vi "Find STM connection by ID.vi"(8 "error in":errorcluster, 10 "Message ID":i32, 11 "STM connections":T1[](array[typedef])) -> (0 "error out":errorcluster, 3 "Connection Ref":T1)   [LabVIEW 2019, in "RemoteControl.STM.lvclass"]
uses:
  RemoteControl.STM.lvclass
  <vilib>/NI/STM/NI STM.lvlib
  <vilib>/NI/STM/TCP/Get Connection Reference (TCP).vi
  <vilib>/NI/STM/SubVIs/MetaDataElement.ctl
  <vilib>/NI/STM/TCP/TCP Connection Info.ctl
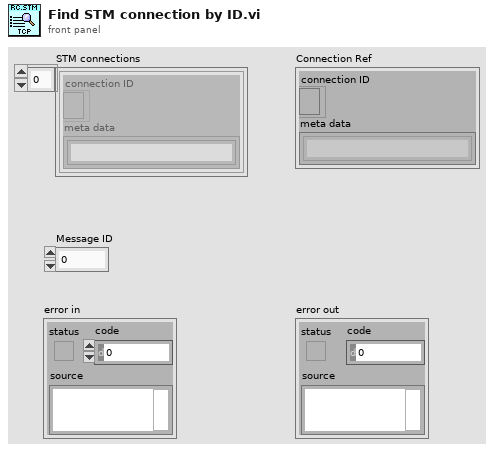
[diagram p1: front panel]
types:
  T1 = typedef "NI STM.lvlib/TCP Connection Info.ctl" = cluster{"connection ID":refnum<k5>, "meta data":T2[]}
  T2 = typedef "NI STM.lvlib/MetaDataElement.ctl" = string
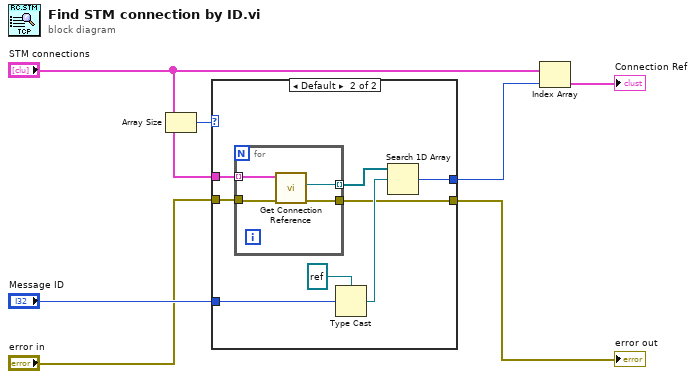
[diagram p0: block diagram]
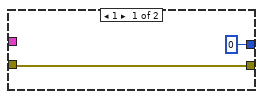
[diagram p2: hidden frame]
diagram:
  n1 = Array Size(array="STM connections") -> (size(s)=w4:i32)
  n2 = case shown="Default" w4 {
    tunnel: "Message ID" -> [_ w15]
    tunnel: "error in" -> [w8 w13]
    tunnel: [w8 w12] -> w5
    tunnel: "STM connections" -> [_ w11]
    tunnel: [0 ("index of element") w10] -> w3
    frame 1 {
    }
    frame Default {
      n3 = for {
        tunnel: w11 -> [w21] mode=indexing
        tunnel: [w20] -> w17 mode=indexing
        tunnel: w13 -> [w19]
        tunnel: [w18] -> w12
        n4 = call-poly <vilib>:"Get Connection Reference.vi"("error in"=w19, "connection info in"=w21) -> ("error out"=w18:errorcluster, "connection ID out"=w20:refnum<k5>)  [unwired: 7 in, 1 out]
      }
      n5 = Type Cast(type=refnum<k5> refnum ("connection ID out"), x=w15) -> (*(type *) &x=w14:refnum<k5>)
      n6 = Search 1D Array(1D array=w17, element=w14) -> (index of element=w10:i32)  [unwired: 1 out]
    }
  }
  "error out" <- w5
  n7 = Index Array(array="STM connections", index=w3) -> (element=→"Connection Ref":T1)
